vi "kuhnke startup debug.vi"() -> ()   [LabVIEW 2019]
uses:
  <vilib>/Platform/TimedLoop/XDataNode/timing_clust.ctl
  <vilib>/Platform/TimedLoop/XDataNode/nitl_modes.ctl
  <vilib>/Platform/TimedLoop/XDataNode/wakeup.ctl
  <vilib>/Utility/file.llb/Read From Spreadsheet File (DBL).vi
  <vilib>/Platform/TimedLoop/XDataNode/XDataNode.xnode
  <vilib>/Platform/TimedLoop/XDataNode/XDNodeRunTimeDep.lvlib
panel:
  in  "Window":i32
  out "Waveform Chart":sgl[][](graph)
  in  "Upper Threshold":dbl=1.0
  out "Starts":u32
  in  "Pos Cross":bool
  in  "Reset":bool
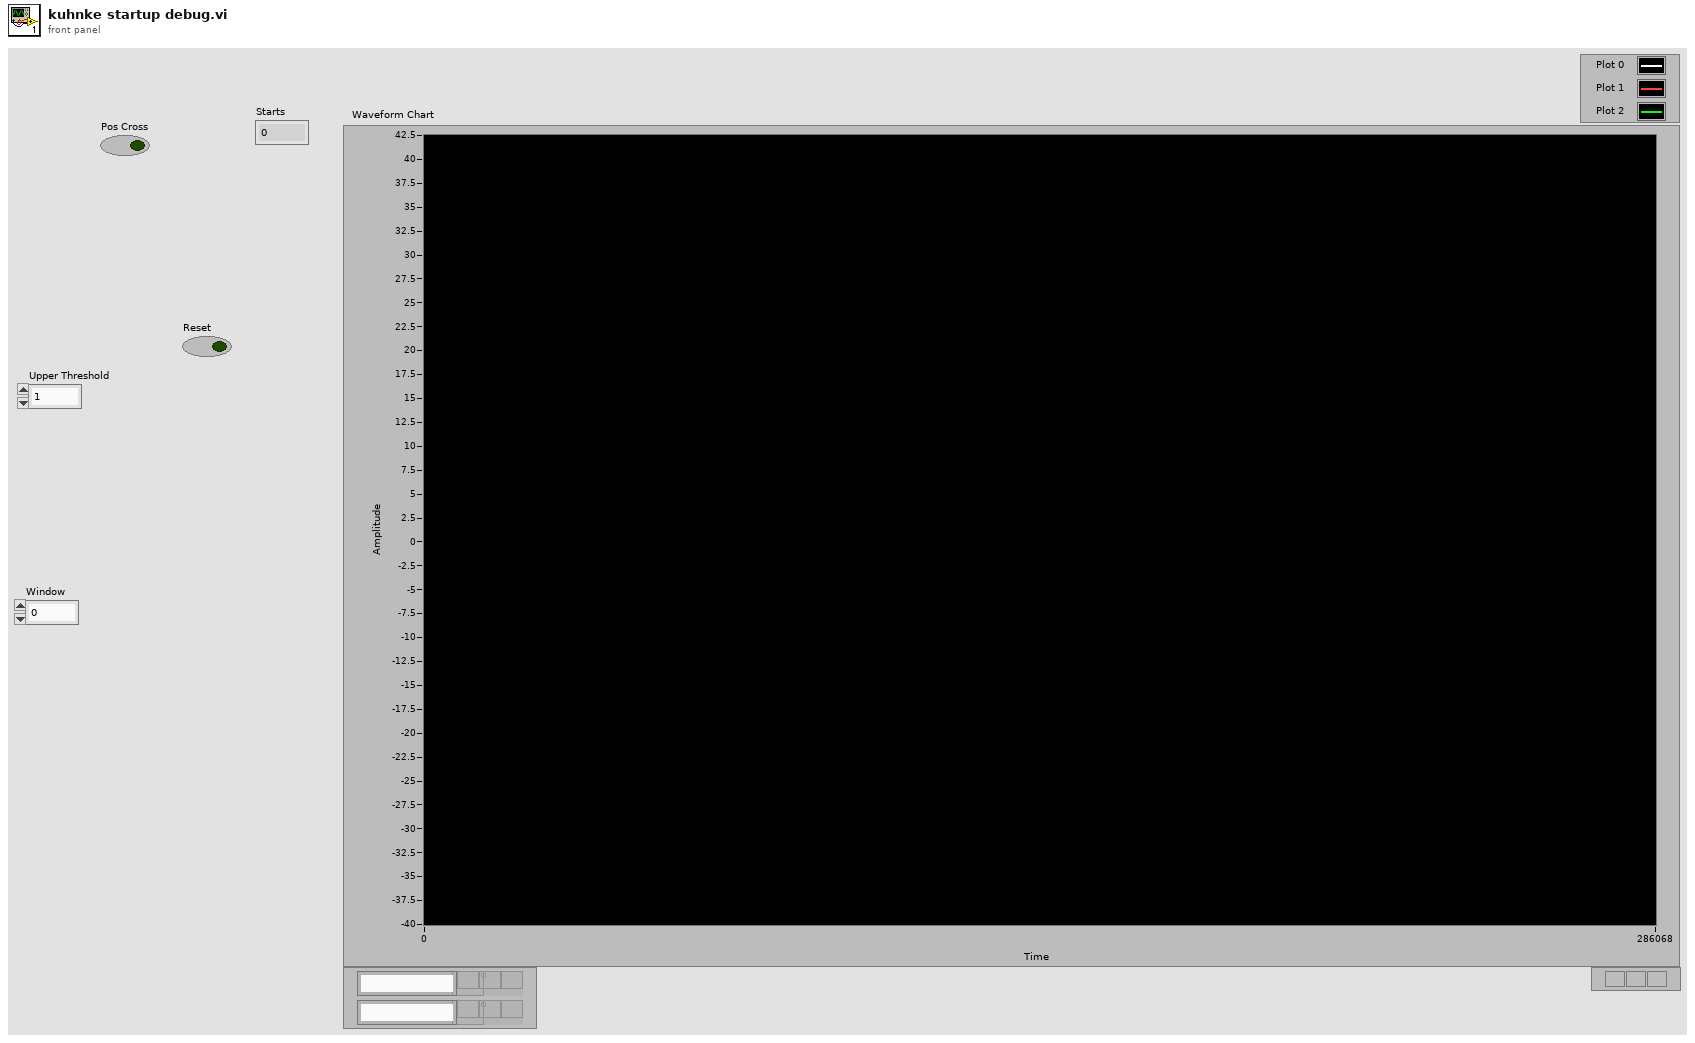
[diagram p1: front panel]
types:
  T1 = typedef "XDNodeRunTimeDep.lvlib/timing_clust.ctl" = cluster{"Expected End [f-1]":u64, "Actual End [f-1]":u64, "Finished Late? [f-1]":bool, "Expected End [i-1]":u64, "Actual End [i-1]":u64, "Finished Late? [i-1]":bool, "Expected Start [i]":u64, "Actual Start [i]":u64, "Expected Start [f]":u64, "Actual Start [f]":u64, "Source Name":string, "Structure Name":string, "Period":i64, "Deadline":i64, "Offset":i64, "Start":i64, "Priority":i32, "Timeout":i32, "Mode":T2, "Wakeup Reason":T3, "Error":errorcluster, "Source Type":string, "Secondary Source Type":string, "Global End Time":u64, "Global Start Time":u64, "Frame Duration":u64, "Iteration Duration":u64, "Assigned CPU":i32, "I/O Scan Engine Mode":u32}
  T2 = typedef "XDNodeRunTimeDep.lvlib/nitl_modes.ctl" = enum32{"No Change", "Process missed periods, maintain original phase", "Discard missed periods, maintain original phase", "Process missed periods, ignore original phase", "Discard missed periods, ignore original phase"}
  T3 = typedef "XDNodeRunTimeDep.lvlib/wakeup.ctl" = enum32{"Normal", "Aborted", "Asynchronous wakeup", "Timing source error", "Timed loop error", "Timeout"}
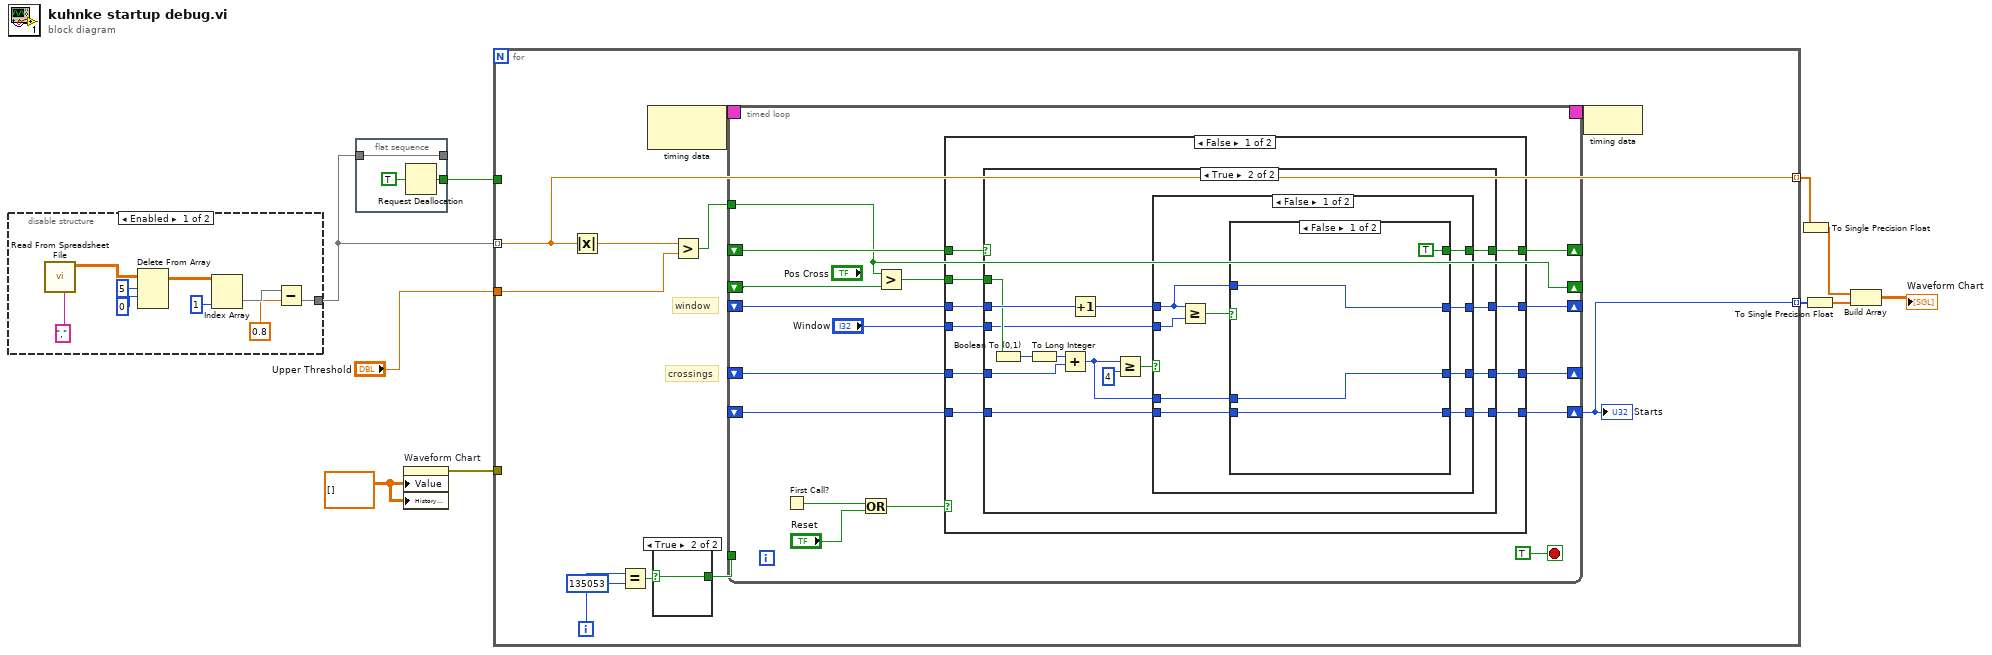
[diagram p0: block diagram]
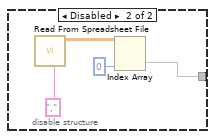
[diagram p2: hidden frame]
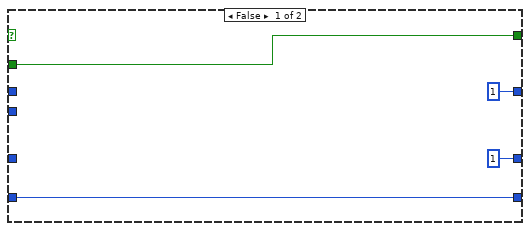
[diagram p4: hidden frame]
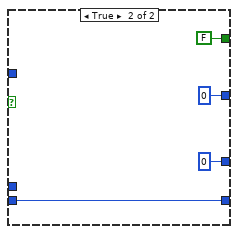
[diagram p5: hidden frame]
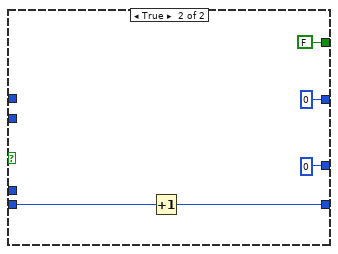
[diagram p6: hidden frame]
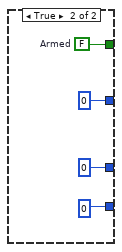
[diagram p7: hidden frame]
diagram:
  w4 = sgl[][] [] ("Waveform Chart")
  n1 = disable-structure shown="Enabled" {
    disable-tunnel: [w11 w20] -> w3
    frame Enabled {
      n2 = call-poly <vilib>:"Read From Spreadsheet File.vi"("delimiter (\\t)"="," ("delimiter (\\t)")) -> ("all rows"=w19:dbl[][])  [unwired: 6 in, 4 out]
      n3 = Delete From Array(array=w19, length=5, index (row)=0) -> (array with subset deleted=w16:dbl[][])  [unwired: 1 in, 1 out]
      n4 = Index Array(array=w16, index (col)=1 ("disabled index (col)")) -> (element=w13:dbl[])  [unwired: 1 in]
      n5 = Subtract(x=w13, y=0.8 ("Upper Threshold")) -> (x-y=w11:dbl[])
    }
    frame Disabled {
      n6 = call-poly <vilib>:"Read From Spreadsheet File.vi"("delimiter (\\t)"="," ("delimiter (\\t)")) -> ("all rows"=w22:dbl[][])  [unwired: 6 in, 4 out]
      n7 = Index Array(array=w22, index (col)=0 ("disabled index (col)")) -> (element=w20:dbl[])  [unwired: 1 in]
    }
  }
  n8 = flat-sequence {
    tunnel: [w25] -> _
    tunnel: w3 -> [w25]
    tunnel: [w24] -> w6
    frame #0 {
      w24 = TRUE ("flag")
      n9 = Request Deallocation(w24) -> ()
    }
  }
  n10 = property on="Waveform Chart" class="WFChart (strict)"("Value"=w4, "History Data"=w4) -> (error out=w5:errorcluster)  [unwired: 2 in, 1 out]
  n11 = for {
    tunnel: [w34] -> w10 mode=indexing
    tunnel: w6 -> [_]
    tunnel: w5 -> [_]
    tunnel: w3 -> [w26] mode=indexing
    tunnel: "Upper Threshold" -> [w33]
    tunnel: [w26] -> w1 mode=indexing
    i -> [w31]
    # "crossings"
    # "window"
    n12 = Absolute Value(x=w26) -> (abs(x)=w27:dbl)
    n13 = Equal?(x=w31, y=135053) -> (x = y?=w29:bool)
    n14 = node-c288() -> (w36:T1)  [unwired: 1 in]
    n15 = case shown="True" w29 {
      selector: w29 -> [w37 w38]
      tunnel: [w37 w38] -> w28
      frame False {
      }
      frame True {
      }
    }
    n16 = Greater?(x=w27, y=w33) -> (0:w32:bool)
    n17 = timed-loop {
      shift-right: [w48] -> w34
      shift-left: _ -> [w49]
      shift-right: [w53] -> _
      shift-left: _ -> [w54]
      shift-right: [w52] -> _
      shift-left: _ -> [w51]
      timing: w36 -> [_]
      timing-out: [_] -> w35
      tunnel: w32 -> [w41]
      tunnel: w28 -> [_]
      shift-right: [w41] -> _
      shift-left: _ -> [w43]
      shift-right: [w40] -> _
      shift-left: _ -> [w39]
      stop <- TRUE stop-if-true
      n18 = First Call?() -> (First Call?: T/F=w47:bool)
      n19 = Or(x=w47, y="Reset") -> (x .or. y?=w46:bool)
      n20 = Greater?(x=w41, y=w43) -> (0:w42:bool)
      n21 = case shown="False" w46 {
        tunnel: w54 -> [w64 _]
        tunnel: [w63 w107] -> w53
        tunnel: [w61 0] -> w52
        tunnel: w51 -> [w59 _]
        tunnel: w49 -> [w57 _]
        tunnel: [w56 u32 0] -> w48
        tunnel: "Window" -> [w55 _]
        tunnel: w42 -> [w62 _]
        tunnel: [w60 0] -> w40
        tunnel: w39 -> [w58 _]
        frame False {
          n22 = case shown="True" w64 {
            tunnel: [w68 w75] -> w63
            tunnel: w62 -> [w68 w82]
            tunnel: [1 ("Window") w74] -> w61
            tunnel: [1 ("Window") w76] -> w60
            tunnel: w59 -> [_ w83]
            tunnel: w58 -> [_ w71]
            tunnel: w57 -> [w65 w78]
            tunnel: [w65 w77] -> w56
            tunnel: w55 -> [_ w72]
            frame False {
            }
            frame True {
              n23 = Boolean To (0,1)(Boolean=w82) -> (0, 1=w81:i16)
              n24 = To Long Integer(number=w81) -> (32bit integer=w69:i32)
              n25 = Add(x=w69, y=w71) -> (x+y=w70:i32)
              n26 = Increment(x=w83) -> (x+1=w73:i32)
              n27 = Greater Or Equal?(x=w70, y=4) -> (x >= y?=w79:bool)
              n28 = case shown="False" w79 {
                tunnel: w78 -> [w90 w105]
                tunnel: [w89 w104] -> w77
                tunnel: [w88 0 ("Window")] -> w76
                tunnel: [w86 FALSE] -> w75
                tunnel: [w87 0 ("Window")] -> w74
                tunnel: w73 -> [w85 _]
                tunnel: w72 -> [w92 _]
                tunnel: w70 -> [w84 _]
                frame False {
                  n29 = Greater Or Equal?(x=w85, y=w92) -> (x >= y?=w91:bool)
                  n30 = case shown="False" w91 {
                    tunnel: [w96 w100] -> w89
                    tunnel: w90 -> [w96 w100]
                    tunnel: [w93 0 ("Window")] -> w88
                    tunnel: [w95 0 ("Window")] -> w87
                    tunnel: [TRUE FALSE] -> w86
                    tunnel: w85 -> [w95 _]
                    tunnel: w84 -> [w93 _]
                    frame False {
                    }
                    frame True {
                    }
                  }
                }
                frame True {
                  n31 = Increment(x=w105) -> (x+1=w104:u32)
                }
              }
            }
          }
        }
        frame True {
          w107 = FALSE  # Armed
        }
      }
    }
    "Starts" <- w34
    n32 = node-c288(w35) -> ()
  }
  n33 = To Single Precision Float(number=w1) -> (single precision float=w8:sgl[])
  n34 = To Single Precision Float(number=w10) -> (single precision float=w9:sgl[])
  n35 = Build Array(w8, w9) -> (→"Waveform Chart":sgl[][])
